vi "Write to File.vi"(8 "error in":errorcluster, 10 "File Actor In":refnum<class "File Actor.lvclass">, 11 "Instr Exe Write to File in":refnum<class "Instr Exe Write to File.lvclass">) -> (0 "error out":errorcluster, 2 "File Actor Out":refnum<class "File Actor.lvclass">)   [LabVIEW 2014, in "Controller.lvlib" / "Instr Exe Write to File.lvclass"]
doc: "This is the sould of the execution method and the only VI that should be overriden. This is where we expect the file to be written."
uses:
  Instr Exe Write to File.lvclass
  File Actor/File Actor.lvclass
  SuperActor/Ex Nested.lvclass/Ex Nested.ctl
  File Actor/File Actor.lvclass/File Actor.ctl
  SuperActor/Read Log Session.vi
  File Actor/Read File DVR.vi
  <userlib>/_Session Fwk/Session - Root.lvclass
  reusable/Session APIs/Session Log/System Log.lvclass
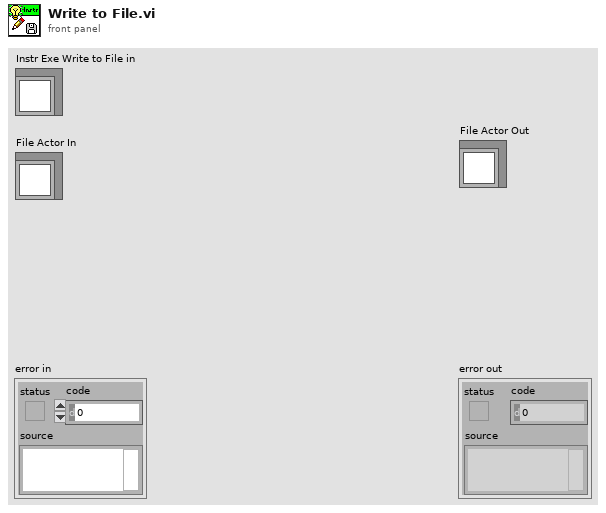
[diagram p1: front panel]
types:
  T1 = typedef "Session - Root.lvclass/Session Handle.ctl" = refnum<data-value>
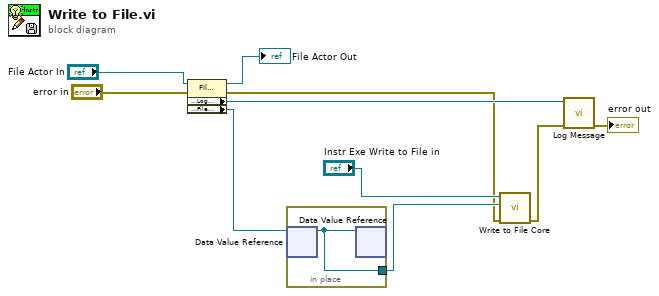
[diagram p0: block diagram]
diagram:
  n1 = property class="File Actor"(reference="File Actor In", error in="error in") -> (reference out=→"File Actor Out":refnum<class "File Actor.lvclass">, error out=w2:errorcluster, "Accessors:Log Session"=w10:T1, "Accessors:File DVR"=w9:refnum<data-value>)
  n2 = in-place {
    in-place-border: [w11] -> w4
    n3 = in-place-dvr #1(w9) -> (w11:refnum<file>)  [unwired: 1 out]
    n4 = in-place-dvr #1(w11) -> ()  [unwired: 2 out]
  }
  n5 = call-dynamic "Write to File Core.vi"("error in (no error)"=w2, "File Ref"=w4, "Instr Exe Write to File in"="Instr Exe Write to File in") -> ("error out"=w1:errorcluster)  [unwired: 7 in, 1 out]
  n6 = call "Log Message.vi"("error in"=w1, "session in"=w10) -> ("error out"=→"error out":errorcluster)  [unwired: 8 in, 1 out]
